vi "Query Calibration kits.vi"(8 "error in (no error)":errorcluster, 10 "Connector type":T1(ring), 11 "VNA-PNA in":refnum<class "VNA-PNA.lvclass">) -> (0 "error out":errorcluster, 2 "Cal kits instaled":string[](array[string]), 3 "VNA-PNA out":refnum<class "VNA-PNA.lvclass">)   [LabVIEW 2020, in "VNA-PNA.lvclass"]
doc: "Queryes the calibration kits installed on the VNA dependent on connector type.\nIf the VNA support E-cal it reports this aswell as the first sting in the array."
uses:
  VNA-PNA.lvclass
  C:/Sandbox/Git_Sandbox/WiSpry Test Framework source code (LV20)/WiSpry Test Framework/Instruments/Instrument.lvclass
  Instrument.lvclass/Instrument.ctl
  Instrument.lvclass
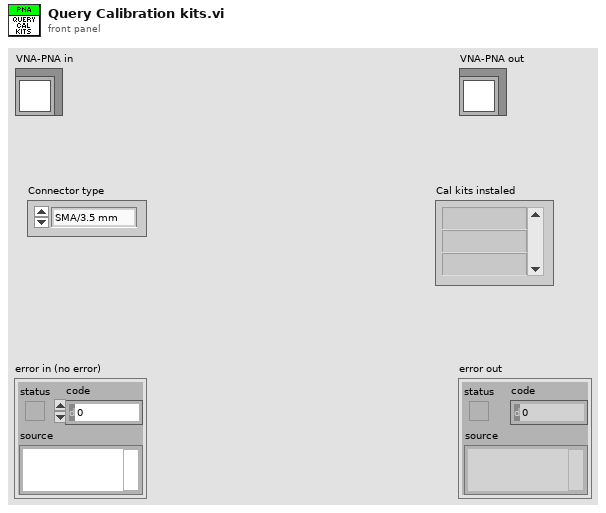
[diagram p1: front panel]
types:
  T1 = enum16{"SMA/3.5 mm", "2.92 mm", "2.4 mm", "1.85 mm", "N 50 Ohm", "N 75 Ohm", "7-16"}
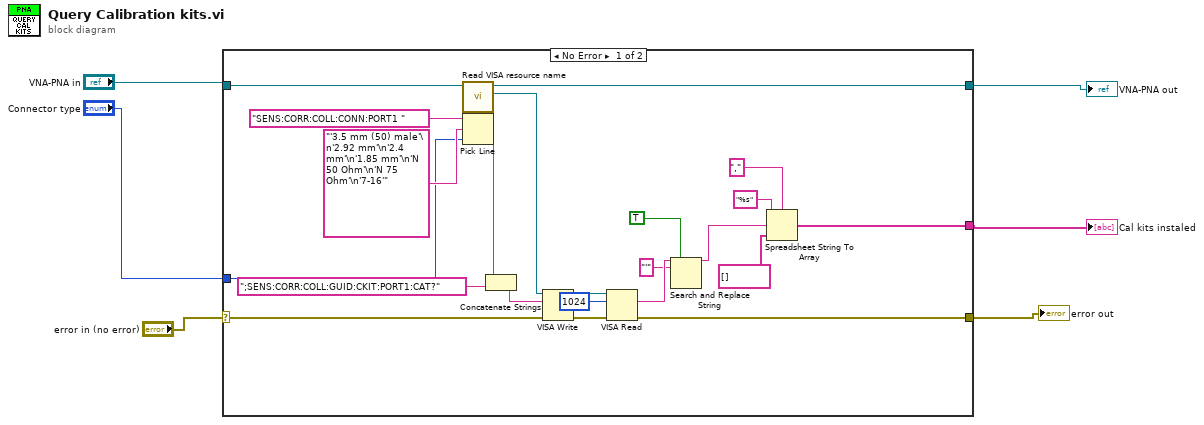
[diagram p0: block diagram]
diagram:
  n1 = case shown="No Error" "error in (no error)" {
    selector: "error in (no error)" -> [w23 w30]
    tunnel: "Connector type" -> [w11 _]
    tunnel: "VNA-PNA in" -> [w28 w29]
    tunnel: [w20 w30] -> w3
    tunnel: [w7 _] -> w2
    tunnel: [w12 w29] -> w1
    frame No Error {
      n2 = call "Read VISA resource name.vi"("Instrument in"=w28) -> ("VISA resource name"=w25:refnum<visa-resource-name>, "Instrument out"=w12:refnum<class "VNA-PNA.lvclass">)  [unwired: 9 in]
      n3 = Pick Line(string ("")="SENS:CORR:COLL:CONN:PORT1 ", multi-line string="'3.5 mm (50) male'\n'2.92 mm'\n'2.4 mm'\n'1.85 mm'\n'N 50 Ohm'\n'N 75 Ohm'\n'7-16'", line index=w11) -> (output string=w24:string)
      n4 = Concatenate Strings(w24, ";SENS:CORR:COLL:GUID:CKIT:PORT1:CAT?" ("string")) -> (w10:string)
      n5 = VISA Write(VISA resource name=w25, write buffer=w10, error in (no error)=w23) -> (VISA resource name out=w21:refnum<visa-resource-name>, error out=w22:errorcluster)  [unwired: 1 out]
      n6 = VISA Read(VISA resource name=w21, byte count=u32 1024, error in (no error)=w22) -> (read buffer=w18:string, error out=w20:errorcluster)  [unwired: 2 out]
      n7 = Search and Replace String(replace all?=TRUE ("replace all? (F)"), input string=w18, search string="'") -> (result string=w15:string)  [unwired: 5 in, 3 out]
      n8 = Spreadsheet String To Array(delimiter (Tab)=",", format string="%s", spreadsheet string=w15, array type (2D Dbl)=string[] [] ("Cal kits instaled")) -> (array=w7:string[])
    }
    frame Error {
    }
  }
  "error out" <- w3
  "VNA-PNA out" <- w1
  "Cal kits instaled" <- w2
